vi "PixyCam_GetByte.vi"(4 "error in":errorcluster, 6 "SendData (T)":bool=TRUE, 7 "PixyCamDevRef":T1) -> (0 "error out":errorcluster, 2 "Word Out":u8, 3 "PixyCamDevRefOut":T1)   [LabVIEW 2016, in "PixyCam_LabVIEW.lvlib"]
uses:
  PixyCam_LabVIEW.lvlib
  PixyCam_DevRef.ctl
  PixyCam_SPI_DevRef.ctl
  <vilib>/Rock Robotics/WPI/SPI/WPI_SPIDevRef.ctl
  <vilib>/Rock Robotics/SystemInterfaces/spilib/spi_bus.ctl
  PixyCam_CommMode.ctl
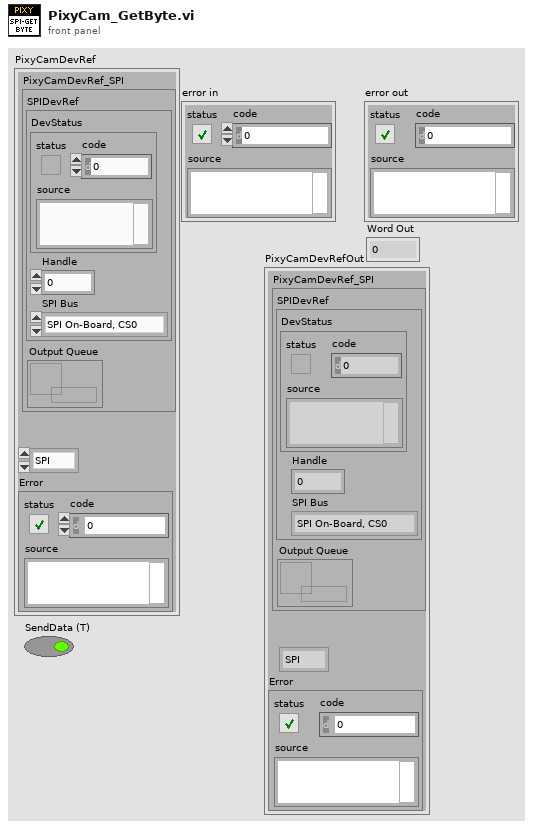
[diagram p1: front panel]
types:
  T1 = typedef "PixyCam_LabVIEW.lvlib/PixyCam_DevRef.ctl" = cluster{"PixyCamDevRef_SPI":T2, "Communication Mode":T5, "Error":errorcluster}
  T2 = typedef "PixyCam_LabVIEW.lvlib/PixyCam_SPI_DevRef.ctl" = cluster{"SPIDevRef":T3, "Output Queue":refnum<queue>}
  T3 = typedef "WPI_SPIDevRef.ctl" = cluster{"DevStatus":errorcluster, "Handle":i32, "SPI Bus":T4}
  T4 = typedef "spi_bus.ctl" = enum16{"SPI On-Board, CS0", "SPI On-Board, CS1", "SPI On-Board, CS2", "SPI On-Board, CS3", "SPI MXP", "Invalid"}
  T5 = typedef "PixyCam_LabVIEW.lvlib/PixyCam_CommMode.ctl" = enum16{"SPI", "I2C", "UART", "Analog", "Digital"}
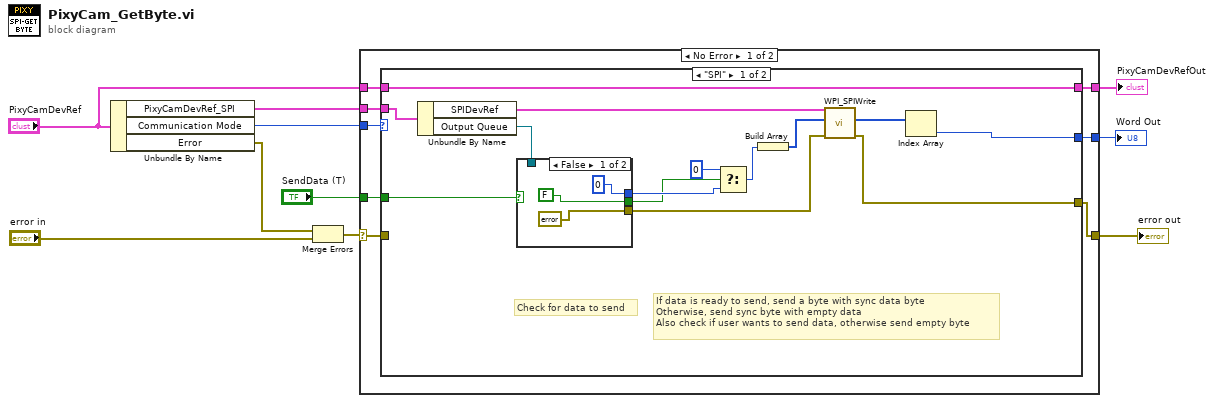
[diagram p0: block diagram]
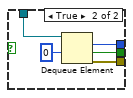
[diagram p2: hidden frame]
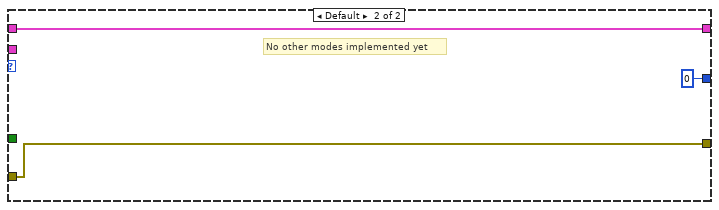
[diagram p3: hidden frame]
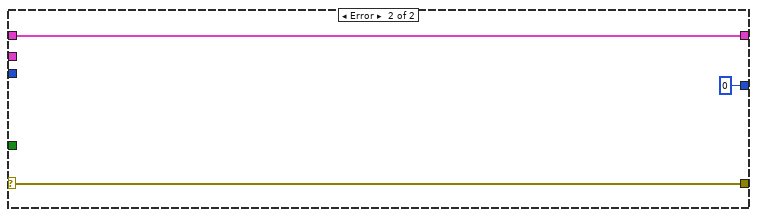
[diagram p4: hidden frame]
diagram:
  n1 = Unbundle By Name("PixyCamDevRef") -> ("PixyCamDevRef_SPI"=w5:T2, "Communication Mode"=w6:T5, "Error"=w10:errorcluster)
  n2 = Merge Errors(w10, "error in") -> (w8:errorcluster)
  n3 = case shown="No Error" w8 {
    selector: w8 -> [w14 w46]
    tunnel: [w15 w46] -> w7
    tunnel: w6 -> [w18 _]
    tunnel: w5 -> [w17 _]
    tunnel: [w16 u16 0] -> w4
    tunnel: [w13 w44] -> w3
    tunnel: "PixyCamDevRef" -> [w12 w44]
    tunnel: "SendData (T)" -> [w11 _]
    frame No Error {
      n4 = case shown="\"SPI\"" w18 {
        tunnel: w17 -> [w32 _]
        tunnel: [w21 u8 0] -> w16
        tunnel: [w24 w43] -> w15
        tunnel: w14 -> [_ w43]
        tunnel: [w22 w41] -> w13
        tunnel: w12 -> [w22 w41]
        tunnel: w11 -> [w19 _]
        frame "SPI" {
          # "Check for data to send"
          # "If data is ready to send, send a byte with sync data byte\nOtherwise, send sync byte with empty data\nAlso check if user wants to send data, otherwise send empty byte"
          n5 = Unbundle By Name(w32) -> ("SPIDevRef"=w30:T3, "Output Queue"=w31:refnum<queue>)
          n6 = case shown="False" w19 {
            tunnel: w31 -> [_ w40]
            tunnel: [u8 0 w38] -> w28
            tunnel: [errorcluster {"status"=FALSE, "code"=0, "source"=""} ("error out") w37] -> w23
            tunnel: [FALSE ("timed out?") w36] -> w20
            frame False {
            }
            frame True {
              n7 = Dequeue Element(queue=w40, timeout in ms (-1)=0) -> (element=w38:u8, timed out?=w36:bool, error out=w37:errorcluster)  [unwired: 1 in, 1 out]
            }
          }
          n8 = Select(t=u8 0, s=w20, f=w28) -> (s? t:f=w26:u8)
          n9 = Build Array(w26) -> (w29:u8[])
          n10 = call <vilib>:"WPI_SPIWrite.vi"("error in (no error)"=w23, "Data To Send"=w29, "SPIDevRef"=w30) -> ("error out"=w24:errorcluster, "Received Data"=w25:u8[])  [unwired: 6 in, 1 out]
          n11 = Index Array(array=w25) -> (element=w21:u8)  [unwired: 1 in]
        }
        frame Default {
          # "No other modes implemented yet"
        }
      }
    }
    frame Error {
    }
  }
  "error out" <- w7
  "Word Out" <- w4
  "PixyCamDevRefOut" <- w3
